vi "Read Helium Meters Remotely.vi"() -> ()   [LabVIEW 2015]
uses:
  Libraries/HeliumMonitor/Sensor configuration.ctl
  Libraries/HeliumMonitor/Channel type.ctl
  <vilib>/Platform/TimedLoop/XDataNode/timing_clust.ctl
  <vilib>/Platform/TimedLoop/XDataNode/nitl_modes.ctl
  <vilib>/Platform/TimedLoop/XDataNode/wakeup.ctl
  <vilib>/platform/TimedLoop/XDataNode/XDataNode.xnode
  <vilib>/Platform/TimedLoop/XDataNode/XDNodeRunTimeDep.lvlib
panel:
  out "Dewar level":i32(slide) scale=0.0..1000.0
  in  "Data Folder":path=path "\\\\eden\\NHMFLDATA/Data/nhmflmonitor/Helium/data"
  in  "Tab Control":T1(tab)
  out "History Graph":T2(graph)
  in  "Sensors":T3[](array[typedef])=[{"Name"="Ghz lab", "URL"="http:\\\\130.55.69.25", "Channels"=[{"type"=enum."Flow meter", "number"=6.0}]}, {"Name"="main bag", "URL"="http:\\\\130.55.69.22", "Channels"=[{"type"=enum."Flow meter", "number"=6.0}, {"type"=enum."Tank pressure", "number"=0.0}, {"type"=enum."Dewar level", "number"=1.0}]}, {"Name"="PPMS 20T", "URL"="http:\\\\130.55.69.42", "Channels"=[{"type"=enum."Flow meter", "number"=6.0}]}]
  out "Communication Status":string[](array[string])
  in  "Ignore errors":bool
  out "Helium tank pressure":dbl(knob) scale=0.0..2000.0
  in  "period (ms)":i32=5000
  in  "Display Graph":bool=TRUE
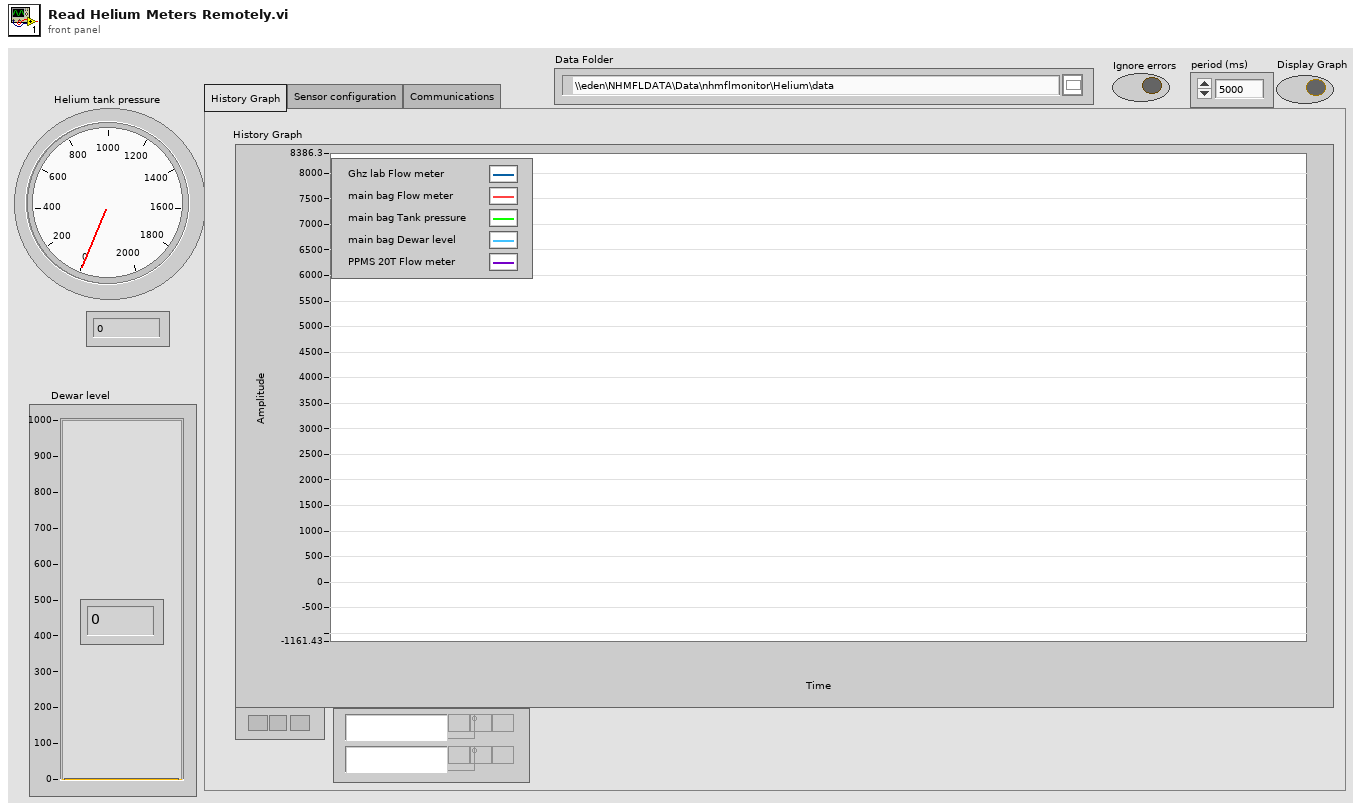
[diagram p1: front panel]
types:
  T1 = enum32{"History Graph", "Sensor configuration", "Communications"}
  T2 = cluster{"output array":dbl[], "output array":dbl[]}[]
  T3 = typedef "Sensor configuration.ctl" = cluster{"Name":string, "URL":string, "Channels":cluster{"type":T4, "number":dbl}[]}
  T4 = typedef "Channel type.ctl" = enum16{"Volts", "Flow meter", "Tank pressure", "Dewar level", "Raw ADC"}
  T5 = typedef "XDNodeRunTimeDep.lvlib/timing_clust.ctl" = cluster{"Expected End [f-1]":u64, "Actual End [f-1]":u64, "Finished Late? [f-1]":bool, "Expected End [i-1]":u64, "Actual End [i-1]":u64, "Finished Late? [i-1]":bool, "Expected Start [i]":u64, "Actual Start [i]":u64, "Expected Start [f]":u64, "Actual Start [f]":u64, "Source Name":string, "Structure Name":string, "Period":i64, "Deadline":i64, "Offset":i64, "Start":i64, "Priority":i32, "Timeout":i32, "Mode":T6, "Wakeup Reason":T7, "Error":errorcluster, "Source Type":string, "Secondary Source Type":string, "Global End Time":u64, "Global Start Time":u64, "Frame Duration":u64, "Iteration Duration":u64, "Assigned CPU":i32, "I/O Scan Engine Mode":u32}
  T6 = typedef "XDNodeRunTimeDep.lvlib/nitl_modes.ctl" = enum32{"No Change", "Process missed periods, maintain original phase", "Discard missed periods, maintain original phase", "Process missed periods, ignore original phase", "Discard missed periods, ignore original phase"}
  T7 = typedef "XDNodeRunTimeDep.lvlib/wakeup.ctl" = enum32{"Normal", "Aborted", "Asynchronous wakeup", "Timing source error", "Timed loop error", "Timeout"}
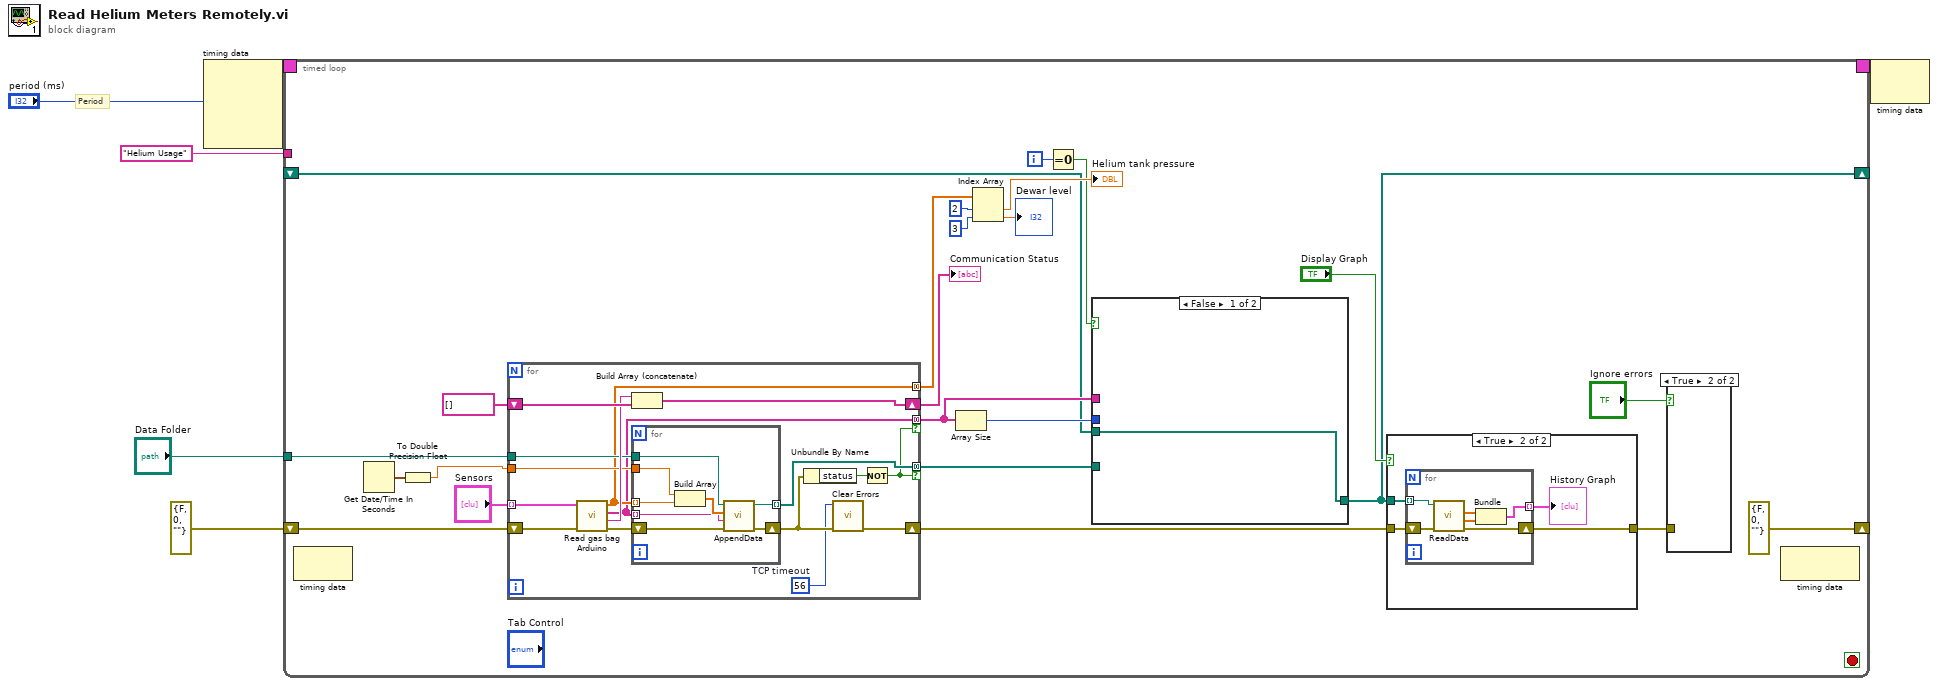
[diagram p0: block diagram]
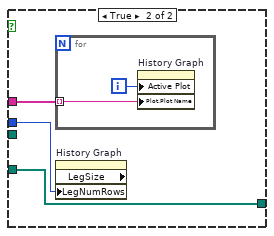
[diagram p2: hidden frame]
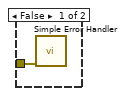
[diagram p3: hidden frame]
diagram:
  # "Period"
  n1 = node-c288("period (ms)") -> (w6:T5)  [unwired: 3 in]
  n2 = timed-loop {
    timing: w6 -> [_]
    timing-out: [_] -> w5
    tunnel: "Data Folder" -> [w15]
    tunnel: "Helium Usage" -> [_]
    shift-right: [errorcluster {"status"=FALSE, "code"=0, "source"=""} ("error out")] -> _
    shift-left: errorcluster {"status"=FALSE, "code"=0, "source"=""} ("error out") -> [w28]
    shift-right: [w7] -> _
    shift-left: _ -> [w8]
    i -> [w20]
    stop <- _ stop-if-true
    n3 = node-c288() -> ()  [unwired: 1 in, 1 out]
    n4 = Get Date/Time In Seconds() -> (seconds since 1Jan1904=w29:timestamp)
    n5 = To Double Precision Float(number=w29) -> (double precision float=w14:dbl)
    n6 = for {
      tunnel: "Sensors" -> [w52] mode=indexing
      shift-right: [w39] -> w13
      shift-left: w28 -> [w53]
      tunnel: [w46] -> w18 mode=concatenating
      tunnel: [w45] -> w11 mode=concatenating if=w41
      shift-right: [w51] -> w16
      shift-left: string[] [] -> [w50]
      tunnel: w15 -> [w48]
      tunnel: w14 -> [w47]
      tunnel: [w42] -> w9 mode=concatenating if=w41
      w38 = 56  # TCP timeout
      n7 = call "Read gas bag Arduino.vi"("Sensor configuration"=w52, "Error In"=w53) -> ("Data"=w46:dbl[], "Names"=w45:string[], "Communication error"=w49:string, "Error Out"=w44:errorcluster)  [unwired: 5 in]
      n8 = Build Array (concatenate)(w49, w50) -> (w51:string[])
      n9 = for {
        shift-right: [w60] -> w40
        shift-left: w44 -> [w59]
        tunnel: w47 -> [w58]
        tunnel: w48 -> [w61]
        tunnel: [w56] -> w42 mode=indexing
        tunnel: w46 -> [w55] mode=indexing
        tunnel: w45 -> [w54] mode=indexing
        n10 = Build Array(w58, w55) -> (w57:dbl[])
        n11 = call "AppendData.vi"("Error In"=w59, "Name"=w54, "Data"=w57, "Folder"=w61) -> ("Error Out"=w60:errorcluster, "File Path Control out"=w56:path)  [unwired: 6 in]
      }
      n12 = Unbundle By Name(w40) -> ("status"=w43:bool)
      n13 = call <vilib>:"Clear Errors.vi"("error in (no error)"=w40, "specific error code to clear (0: all)"=w38) -> ("error out"=w39:errorcluster)  [unwired: 4 in, 1 out]
      n14 = Not(x=w43) -> (.not. x?=w41:bool)
    }
    "Communication Status" <- w16
    n15 = Array Size(array=w11) -> (size(s)=w12:i32)
    n16 = Index Array(array=w18, index #1=2 ("index"), index #2=3 ("index")) -> (element #1=→"Helium tank pressure":dbl, element #2=→"Dewar level":dbl)
    n17 = Equal To 0?(x=w20) -> (x = 0?=w10:bool)
    n18 = case shown="False" w10 {
      tunnel: w11 -> [_ w34]
      tunnel: w12 -> [_ w33]
      tunnel: w9 -> [_ w32]
      tunnel: [w31 w32] -> w7
      tunnel: w8 -> [w31 _]
      frame False {
      }
      frame True {
        n19 = for {
          tunnel: w34 -> [w36] mode=indexing
          i -> [w35]
          n20 = property on="History Graph" class="XYGraph (strict)"("Active Plot"=w35, "Plot.Plot Name"=w36) -> ()  [unwired: 2 in, 2 out]
        }
        n21 = property on="History Graph" class="XYGraph (strict)" props=["LegSize", "LegNumRows"]("LegNumRows"=w33) -> ()  [unwired: 2 in, 3 out]
      }
    }
    n22 = case shown="True" "Display Graph" {
      tunnel: w7 -> [_ w63]
      tunnel: w13 -> [w62 w66]
      tunnel: [w62 w65] -> w26
      frame False {
      }
      frame True {
        n23 = for {
          shift-right: [w71] -> w65
          shift-left: w66 -> [w72]
          tunnel: [w70] -> w64 mode=indexing
          tunnel: w63 -> [w67] mode=indexing
          n24 = call "ReadData.vi"("Error In"=w72, "File Path Control"=w67) -> ("Error Out"=w71:errorcluster, "Y"=w68:dbl[], "X"=w69:dbl[])  [unwired: 6 in, 1 out]
          n25 = Bundle("X"=w69, "Y"=w68) -> (w70:cluster{"X":dbl[], "Y":dbl[]})  [unwired: 1 in]
        }
        "History Graph" <- w64
      }
    }
    n26 = case shown="True" "Ignore errors" {
      tunnel: w26 -> [w37 _]
      frame False {
        n27 = call <vilib>:"Simple Error Handler.vi"("error in (no error)"=w37) -> ()  [unwired: 4 in, 5 out]
      }
      frame True {
      }
    }
    n28 = node-c288() -> ()  [unwired: 1 in, 1 out]
  }
  n29 = node-c288(w5) -> ()  [unwired: 1 out]
